vi "Encoders 1 SUBVI.vi"   [LabVIEW 2011]
uses:
  Robot Global Data.vi
types:
  T1 = typedef "WPI_RobotDriveDevRef.ctl" = cluster{"DevStatus":errorcluster, "Motors[]":T2[], "Square Inputs":bool, "Max Output":dbl, "Isochronous":bool}
  T2 = typedef "WPI_MotorControlDeviceRef.ctl" = cluster{"DeviceStatus":errorcluster, "Type":enum16{"PWM", "CAN"}, "PWM":cluster{"Digital Module":T3, "PWM Channel":T4, "DeadBand":T5}, "CAN":cluster{"Device Number":u8, "Control Mode":T6, "Semaphore":T7, "Max Vout":dbl}, "Invert":bool, "TransformRef":T8, "InvTransformRef":T8}
  T3 = typedef "FPGA_TypedefDigitalModule.ctl" = enum16{"Digital Module 1", "Digital Module 2"}
  T4 = typedef "FPGA_DIOPWMChannel.ctl" = enum8{"PWM 1", "PWM 2", "PWM 3", "PWM 4", "PWM 5", "PWM 6", "PWM 7", "PWM 8", "PWM 9", "PWM 10", "Invalid"}
  T5 = typedef "WPI_PWMDeadband.ctl" = cluster{"Name":string, "maxPositivePwm":i32, "minPositivePwm":i32, "centerPwm":i32, "maxNegativePwm":i32, "minNegativePwm":i32, "angularRange":u16}
  T6 = typedef "WPI_CANJaguar_ControlMode.ctl" = enum8{"Percent VBus", "Current", "Speed", "Position", "Voltage"}
  T7 = typedef "Semaphore RefNum" = refnum<k1>
  T8 = typedef "WPI_PWMTransform_ConPane.ctl" = refnum<vi>
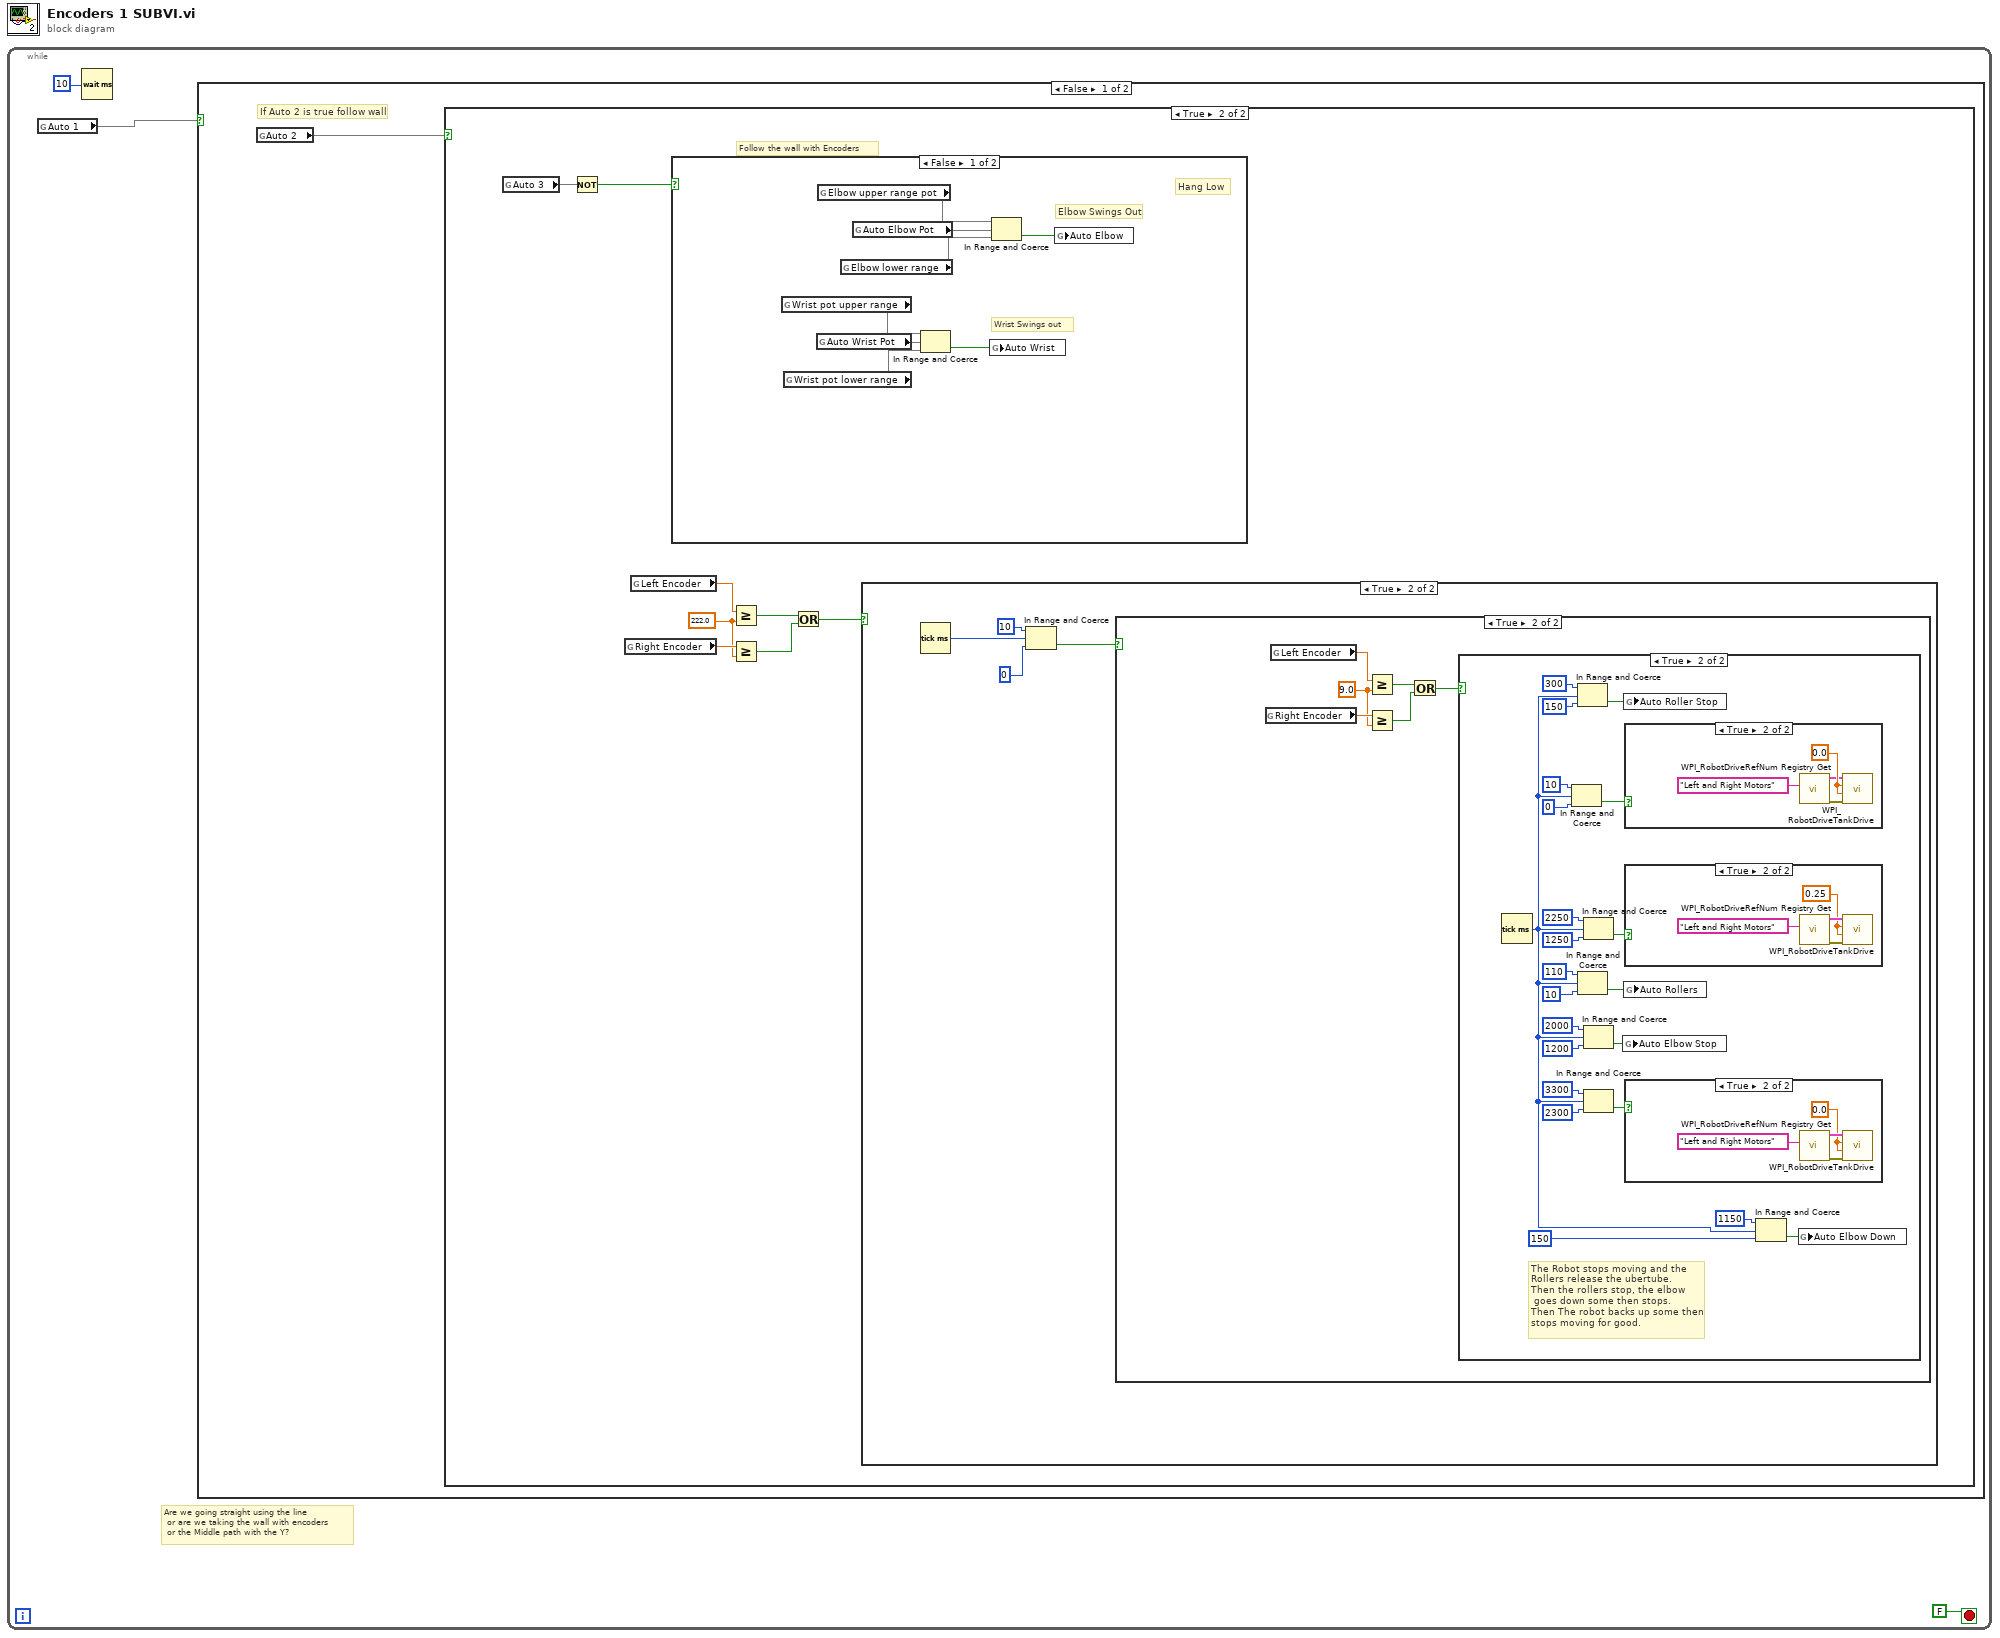
[diagram p0: block diagram]
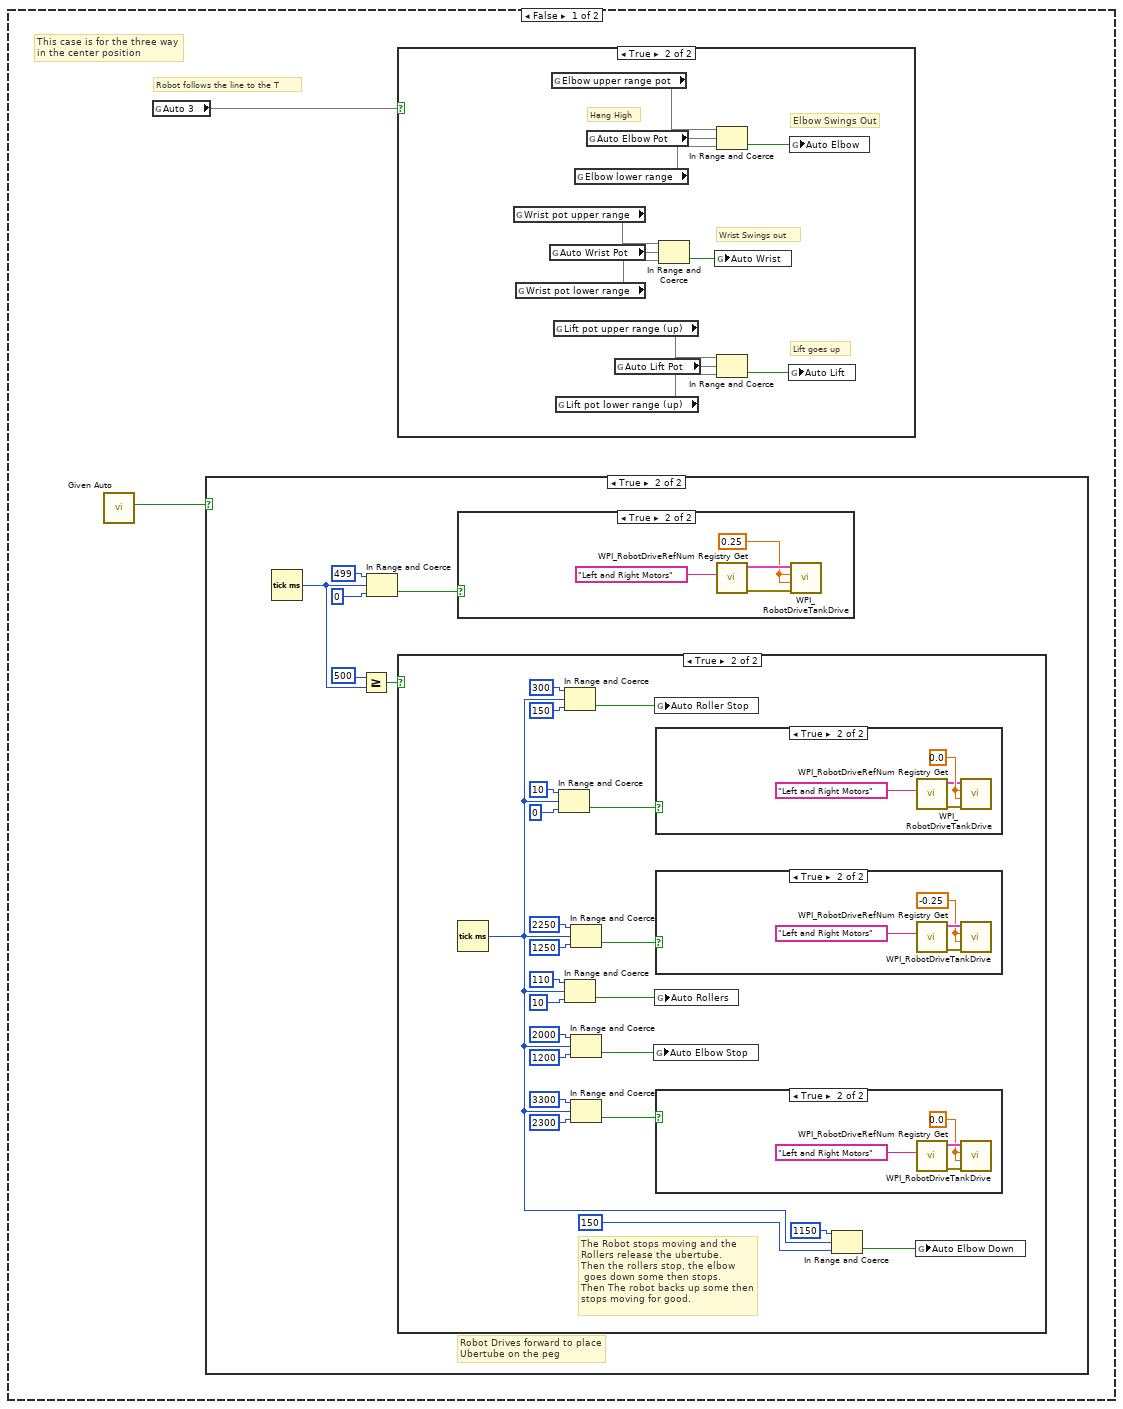
[diagram p2: hidden frame]
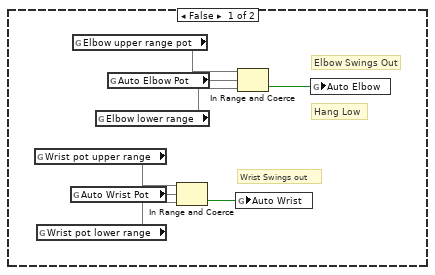
[diagram p9: hidden frame]
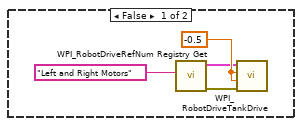
[diagram p10: hidden frame]
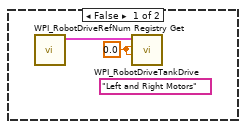
[diagram p11: hidden frame]
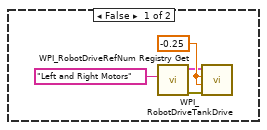
[diagram p12: hidden frame]
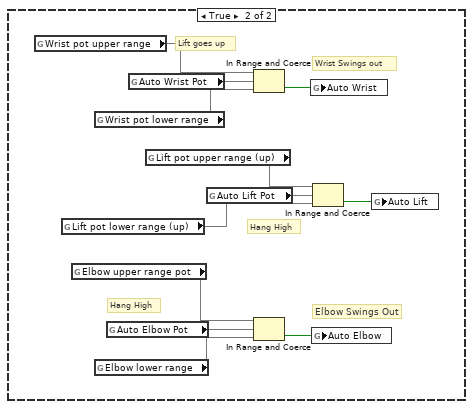
[diagram p16: hidden frame]
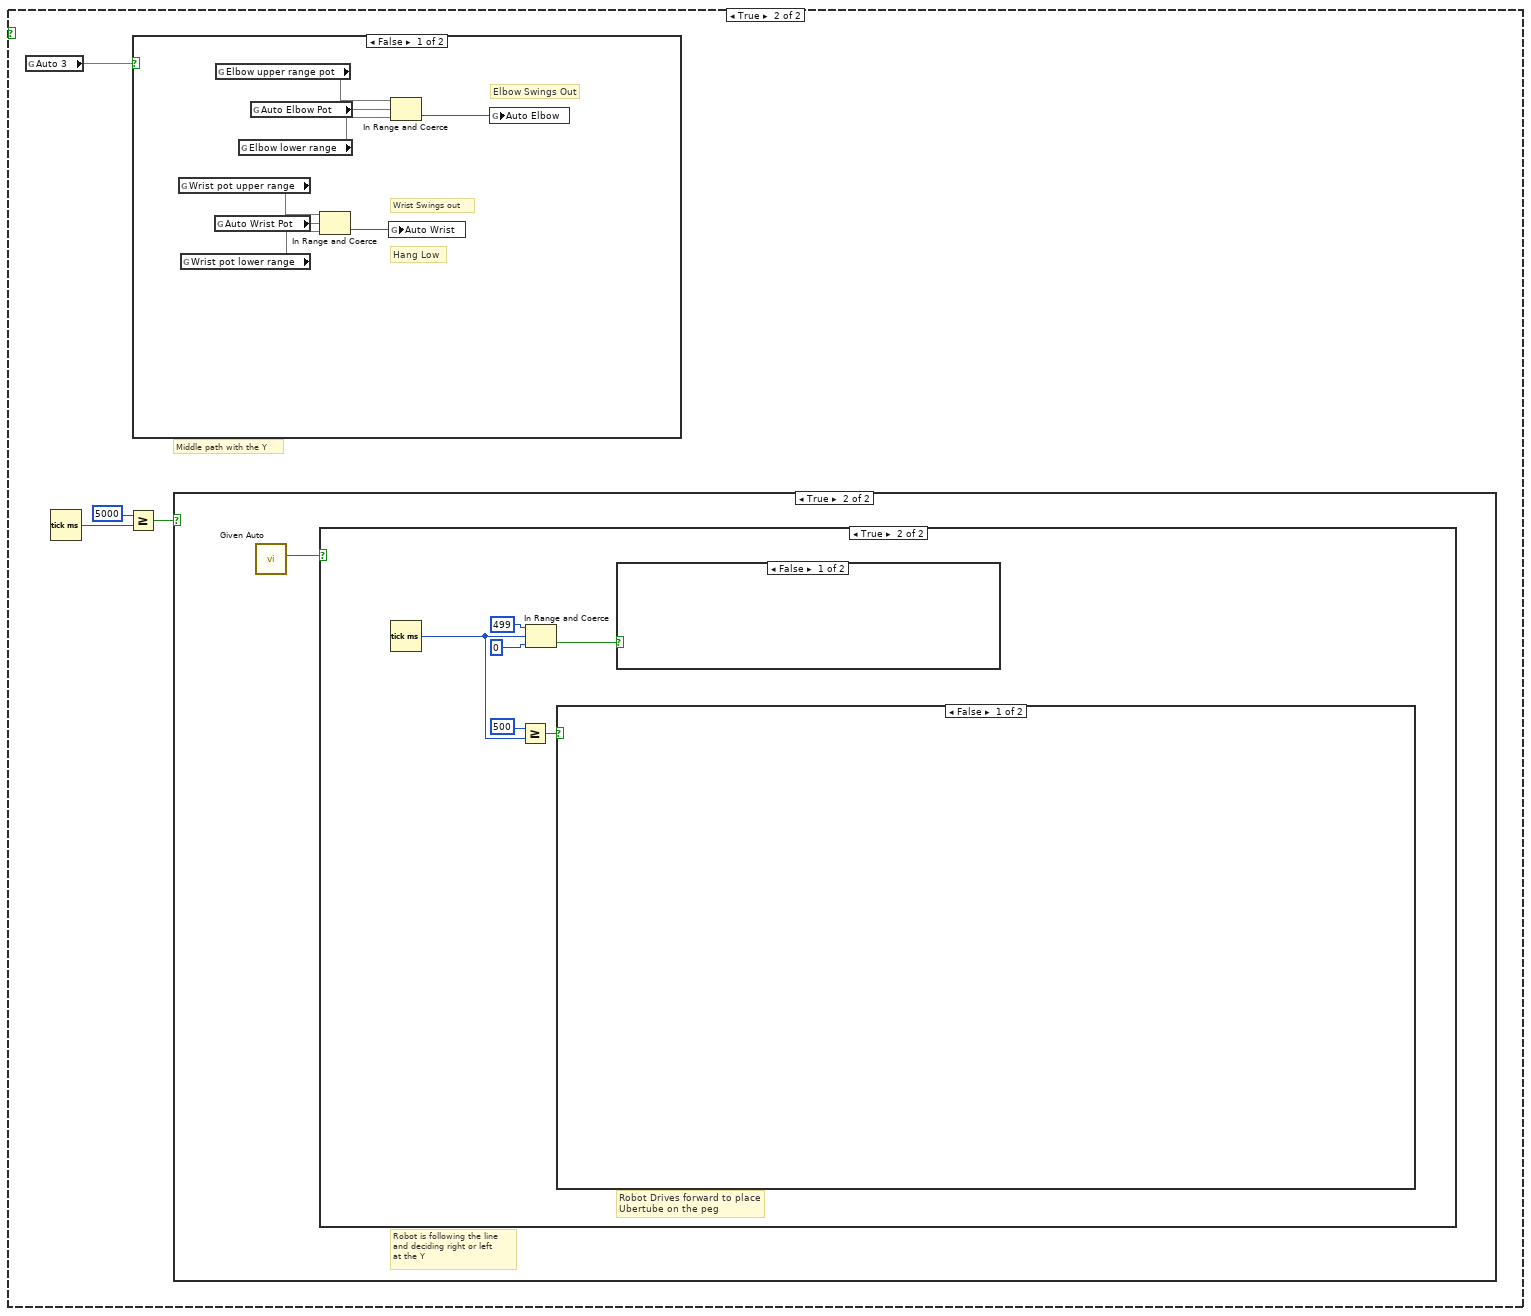
[diagram p17: hidden frame]
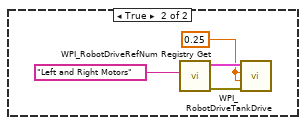
[diagram p20: hidden frame]
diagram:
  n1 = while {
    stop <- FALSE stop-if-true
    # "Are we going straight using the line\n or are we taking the wall with encoders\n or the Middle path with the Y?"
    n2 = global read "Robot Global Data.vi" "Auto 1"() -> (w1)
    n3 = Wait (ms)(milliseconds to wait=u32 10) -> ()  [unwired: 1 out]
    n4 = case shown="False" w1 {
      frame False {
        # "If Auto 2 is true follow wall"
        n5 = global read "Robot Global Data.vi" "Auto 2"() -> (w4)
        n6 = case shown="True" w4 {
          frame False {
            # "Robot follows the line to the T"
            # "This case is for the three way \nin the center position"
            n7 = call "Given Auto.vi"() -> ("x .or. y?"=w6:bool)  [unwired: 11 out]
            n8 = global read "Robot Global Data.vi" "Auto 3"() -> (w5)
            n9 = case shown="True" w6 {
              frame False {
              }
              frame True {
                # "Robot Drives forward to place\nUbertube on the peg"
                n10 = Tick Count (ms)() -> (millisecond timer value=w9:u32)
                n11 = Greater Or Equal?(x=u32 500, y=w9) -> (x >= y?=w11:bool)
                n12 = In Range and Coerce(upper limit=u32 499, x=w9, lower limit=u32 0) -> (In Range?=w10:bool)  [unwired: 1 out]
                n13 = case shown="True" w11 {
                  frame False {
                  }
                  frame True {
                    # "The Robot stops moving and the \nRollers release the ubertube. \nThen the rollers stop, the elbow\n goes down some then stops. \nThen The robot backs up some then \nstops moving for good."
                    n14 = Tick Count (ms)() -> (millisecond timer value=w17:u32)
                    n15 = In Range and Coerce(upper limit=u32 10, x=w17, lower limit=u32 0 ("x")) -> (In Range?=w18:bool)  [unwired: 1 out]
                    n16 = In Range and Coerce(upper limit=u32 300, x=w17, lower limit=u32 150 ("x")) -> (In Range?=w36:bool)  [unwired: 1 out]
                    n17 = In Range and Coerce(upper limit=u32 110, x=w17, lower limit=u32 10 ("x")) -> (In Range?=w38:bool)  [unwired: 1 out]
                    n18 = In Range and Coerce(upper limit=u32 2250, x=w17, lower limit=u32 1250 ("x")) -> (In Range?=w34:bool)  [unwired: 1 out]
                    n19 = In Range and Coerce(upper limit=u32 2000, x=w17, lower limit=u32 1200) -> (In Range?=w35:bool)  [unwired: 1 out]
                    n20 = In Range and Coerce(upper limit=u32 3300, x=w17, lower limit=u32 2300 ("x")) -> (In Range?=w33:bool)  [unwired: 1 out]
                    n21 = global write "Robot Global Data.vi" "Auto Elbow Stop"(w35) -> ()
                    n22 = global write "Robot Global Data.vi" "Auto Roller Stop"(w36) -> ()
                    n23 = global write "Robot Global Data.vi" "Auto Rollers"(w38) -> ()
                    n24 = case shown="True" w18 {
                      frame False {
                      }
                      frame True {
                        w42 = 0.0 ("Left axis value")
                        n25 = call <vilib>:"WPI_RobotDriveRefNum Registry Get.vi"("refnum name"="Left and Right Motors") -> ("error out"=w40:errorcluster, "RobotDriveDevRef"=w41:T1)  [unwired: 1 in, 8 out]
                        n26 = call <vilib>:"WPI_RobotDriveTankDrive.vi"("error in (no error)"=w40, "Right axis value"=w42, "Left axis value"=w42, "RobotDriveDevRef"=w41) -> ()  [unwired: 8 out]
                      }
                    }
                    n27 = case shown="True" w34 {
                      frame False {
                      }
                      frame True {
                        w47 = -0.25 ("Left axis value")
                        n28 = call <vilib>:"WPI_RobotDriveRefNum Registry Get.vi"("refnum name"="Left and Right Motors") -> ("error out"=w49:errorcluster, "RobotDriveDevRef"=w48:T1)  [unwired: 1 in, 8 out]
                        n29 = call <vilib>:"WPI_RobotDriveTankDrive.vi"("error in (no error)"=w49, "Right axis value"=w47, "Left axis value"=w47, "RobotDriveDevRef"=w48) -> ()  [unwired: 8 out]
                      }
                    }
                    n30 = case shown="True" w33 {
                      frame False {
                      }
                      frame True {
                        w43 = 0.0 ("Left axis value")
                        n31 = call <vilib>:"WPI_RobotDriveRefNum Registry Get.vi"("refnum name"="Left and Right Motors") -> ("error out"=w45:errorcluster, "RobotDriveDevRef"=w44:T1)  [unwired: 1 in, 8 out]
                        n32 = call <vilib>:"WPI_RobotDriveTankDrive.vi"("error in (no error)"=w45, "Right axis value"=w43, "Left axis value"=w43, "RobotDriveDevRef"=w44) -> ()  [unwired: 8 out]
                      }
                    }
                    n33 = In Range and Coerce(upper limit=u32 1150, x=w17, lower limit=u32 150 ("x")) -> (In Range?=w37:bool)  [unwired: 1 out]
                    n34 = global write "Robot Global Data.vi" "Auto Elbow Down"(w37) -> ()
                  }
                }
                n35 = case shown="True" w10 {
                  frame False {
                  }
                  frame True {
                    w13 = 0.25 ("Left axis value")
                    n36 = call <vilib>:"WPI_RobotDriveRefNum Registry Get.vi"("refnum name"="Left and Right Motors") -> ("error out"=w15:errorcluster, "RobotDriveDevRef"=w14:T1)  [unwired: 1 in, 8 out]
                    n37 = call <vilib>:"WPI_RobotDriveTankDrive.vi"("error in (no error)"=w15, "Right axis value"=w13, "Left axis value"=w13, "RobotDriveDevRef"=w14) -> ()  [unwired: 8 out]
                  }
                }
              }
            }
            n38 = case shown="True" w5 {
              frame False {
                # "Elbow Swings Out"
                # "Wrist Swings out"
                # "Hang Low"
                n39 = global read "Robot Global Data.vi" "Wrist pot upper range"() -> (w52)
                n40 = global read "Robot Global Data.vi" "Wrist pot lower range"() -> (w51)
                n41 = global read "Robot Global Data.vi" "Auto Wrist Pot"() -> (w57)
                n42 = global read "Robot Global Data.vi" "Elbow upper range pot"() -> (w54)
                n43 = global read "Robot Global Data.vi" "Elbow lower range"() -> (w53)
                n44 = global read "Robot Global Data.vi" "Auto Elbow Pot"() -> (w55)
                n45 = In Range and Coerce(upper limit=w52, x=w57, lower limit=w51) -> (In Range?=w58:bool)  [unwired: 1 out]
                n46 = global write "Robot Global Data.vi" "Auto Wrist"(w58) -> ()
                n47 = In Range and Coerce(upper limit=w54, x=w55, lower limit=w53) -> (In Range?=w56:bool)  [unwired: 1 out]
                n48 = global write "Robot Global Data.vi" "Auto Elbow"(w56) -> ()
              }
              frame True {
                # "Wrist Swings out"
                # "Elbow Swings Out"
                # "Lift goes up"
                # "Hang High"
                n49 = global read "Robot Global Data.vi" "Wrist pot upper range"() -> (w62)
                n50 = global read "Robot Global Data.vi" "Wrist pot lower range"() -> (w61)
                n51 = global read "Robot Global Data.vi" "Auto Wrist Pot"() -> (w66)
                n52 = global read "Robot Global Data.vi" "Elbow upper range pot"() -> (w60)
                n53 = global read "Robot Global Data.vi" "Lift pot upper range (up)"() -> (w64)
                n54 = global read "Robot Global Data.vi" "Lift pot lower range (up)"() -> (w63)
                n55 = global read "Robot Global Data.vi" "Elbow lower range"() -> (w59)
                n56 = global read "Robot Global Data.vi" "Auto Elbow Pot"() -> (w69)
                n57 = global read "Robot Global Data.vi" "Auto Lift Pot"() -> (w70)
                n58 = In Range and Coerce(upper limit=w62, x=w66, lower limit=w61) -> (In Range?=w65:bool)  [unwired: 1 out]
                n59 = global write "Robot Global Data.vi" "Auto Wrist"(w65) -> ()
                n60 = In Range and Coerce(upper limit=w60, x=w69, lower limit=w59) -> (In Range?=w68:bool)  [unwired: 1 out]
                n61 = In Range and Coerce(upper limit=w64, x=w70, lower limit=w63) -> (In Range?=w67:bool)  [unwired: 1 out]
                n62 = global write "Robot Global Data.vi" "Auto Lift"(w67) -> ()
                n63 = global write "Robot Global Data.vi" "Auto Elbow"(w68) -> ()
              }
            }
          }
          frame True {
            w74 = 222.0 ("y")
            # "Follow the wall with Encoders"
            n64 = global read "Robot Global Data.vi" "Auto 3"() -> (w78)
            n65 = Not(x=w78) -> (.not. x?=w77:bool)
            n66 = global read "Robot Global Data.vi" "Right Encoder"() -> (w75:dbl)
            n67 = global read "Robot Global Data.vi" "Left Encoder"() -> (w76:dbl)
            n68 = case shown="False" w77 {
              frame False {
                # "Elbow Swings Out"
                # "Wrist Swings out"
                # "Hang Low"
                n69 = global read "Robot Global Data.vi" "Wrist pot upper range"() -> (w134)
                n70 = global read "Robot Global Data.vi" "Wrist pot lower range"() -> (w133)
                n71 = global read "Robot Global Data.vi" "Auto Wrist Pot"() -> (w139)
                n72 = global read "Robot Global Data.vi" "Elbow upper range pot"() -> (w136)
                n73 = global read "Robot Global Data.vi" "Elbow lower range"() -> (w135)
                n74 = global read "Robot Global Data.vi" "Auto Elbow Pot"() -> (w137)
                n75 = In Range and Coerce(upper limit=w134, x=w139, lower limit=w133) -> (In Range?=w140:bool)  [unwired: 1 out]
                n76 = global write "Robot Global Data.vi" "Auto Wrist"(w140) -> ()
                n77 = In Range and Coerce(upper limit=w136, x=w137, lower limit=w135) -> (In Range?=w138:bool)  [unwired: 1 out]
                n78 = global write "Robot Global Data.vi" "Auto Elbow"(w138) -> ()
              }
              frame True {
                # "Hang High"
                # "Wrist Swings out"
                # "Elbow Swings Out"
                # "Lift goes up"
                # "Hang High"
                n79 = global read "Robot Global Data.vi" "Wrist pot upper range"() -> (w144)
                n80 = global read "Robot Global Data.vi" "Lift pot lower range (up)"() -> (w141)
                n81 = global read "Robot Global Data.vi" "Elbow upper range pot"() -> (w146)
                n82 = global read "Robot Global Data.vi" "Wrist pot lower range"() -> (w143)
                n83 = global read "Robot Global Data.vi" "Elbow lower range"() -> (w145)
                n84 = global read "Robot Global Data.vi" "Auto Elbow Pot"() -> (w151)
                n85 = global read "Robot Global Data.vi" "Auto Wrist Pot"() -> (w148)
                n86 = global read "Robot Global Data.vi" "Lift pot upper range (up)"() -> (w142)
                n87 = global read "Robot Global Data.vi" "Auto Lift Pot"() -> (w152)
                n88 = In Range and Coerce(upper limit=w144, x=w148, lower limit=w143) -> (In Range?=w147:bool)  [unwired: 1 out]
                n89 = In Range and Coerce(upper limit=w146, x=w151, lower limit=w145) -> (In Range?=w150:bool)  [unwired: 1 out]
                n90 = global write "Robot Global Data.vi" "Auto Wrist"(w147) -> ()
                n91 = global write "Robot Global Data.vi" "Auto Elbow"(w150) -> ()
                n92 = In Range and Coerce(upper limit=w142, x=w152, lower limit=w141) -> (In Range?=w149:bool)  [unwired: 1 out]
                n93 = global write "Robot Global Data.vi" "Auto Lift"(w149) -> ()
              }
            }
            n94 = Greater Or Equal?(x=w76, y=w74) -> (x >= y?=w73:bool)
            n95 = Greater Or Equal?(x=w75, y=w74) -> (x >= y?=w72:bool)
            n96 = Or(x=w73, y=w72) -> (x .or. y?=w71:bool)
            n97 = case shown="True" w71 {
              frame False {
                w82 = -0.5 ("Left axis value")
                n98 = call <vilib>:"WPI_RobotDriveRefNum Registry Get.vi"("refnum name"="Left and Right Motors") -> ("error out"=w80:errorcluster, "RobotDriveDevRef"=w81:T1)  [unwired: 1 in, 8 out]
                n99 = call <vilib>:"WPI_RobotDriveTankDrive.vi"("error in (no error)"=w80, "Right axis value"=w82, "Left axis value"=w82, "RobotDriveDevRef"=w81) -> ()  [unwired: 8 out]
              }
              frame True {
                n100 = Tick Count (ms)() -> (millisecond timer value=w83:u32)
                n101 = In Range and Coerce(upper limit=u32 10, x=w83, lower limit=u32 0 ("millisecond timer value")) -> (In Range?=w85:bool)  [unwired: 1 out]
                n102 = case shown="True" w85 {
                  frame False {
                    w87 = 0.0 ("Left axis value")
                    (unwired) "Left and Right Motors" ("refnum name")
                    n103 = call <vilib>:"WPI_RobotDriveRefNum Registry Get.vi"() -> ("RobotDriveDevRef"=w88:T1)  [unwired: 2 in, 9 out]
                    n104 = call <vilib>:"WPI_RobotDriveTankDrive.vi"("Right axis value"=w87, "Left axis value"=w87, "RobotDriveDevRef"=w88) -> ()  [unwired: 1 in, 8 out]
                  }
                  frame True {
                    w92 = 9.0 ("y")
                    n105 = global read "Robot Global Data.vi" "Right Encoder"() -> (w93:dbl)
                    n106 = global read "Robot Global Data.vi" "Left Encoder"() -> (w94:dbl)
                    n107 = Greater Or Equal?(x=w94, y=w92) -> (x >= y?=w91:bool)
                    n108 = Greater Or Equal?(x=w93, y=w92) -> (x >= y?=w90:bool)
                    n109 = Or(x=w91, y=w90) -> (x .or. y?=w89:bool)
                    n110 = case shown="True" w89 {
                      frame False {
                        w98 = -0.25 ("Left axis value")
                        n111 = call <vilib>:"WPI_RobotDriveRefNum Registry Get.vi"("refnum name"="Left and Right Motors") -> ("error out"=w96:errorcluster, "RobotDriveDevRef"=w97:T1)  [unwired: 1 in, 8 out]
                        n112 = call <vilib>:"WPI_RobotDriveTankDrive.vi"("error in (no error)"=w96, "Right axis value"=w98, "Left axis value"=w98, "RobotDriveDevRef"=w97) -> ()  [unwired: 8 out]
                      }
                      frame True {
                        # "The Robot stops moving and the \nRollers release the ubertube. \nThen the rollers stop, the elbow\n goes down some then stops. \nThen The robot backs up some then \nstops moving for good."
                        n113 = Tick Count (ms)() -> (millisecond timer value=w99:u32)
                        n114 = In Range and Coerce(upper limit=u32 10, x=w99, lower limit=u32 0 ("x")) -> (In Range?=w100:bool)  [unwired: 1 out]
                        n115 = In Range and Coerce(upper limit=u32 300, x=w99, lower limit=u32 150 ("x")) -> (In Range?=w118:bool)  [unwired: 1 out]
                        n116 = In Range and Coerce(upper limit=u32 110, x=w99, lower limit=u32 10 ("x")) -> (In Range?=w120:bool)  [unwired: 1 out]
                        n117 = In Range and Coerce(upper limit=u32 2250, x=w99, lower limit=u32 1250 ("x")) -> (In Range?=w116:bool)  [unwired: 1 out]
                        n118 = In Range and Coerce(upper limit=u32 2000, x=w99, lower limit=u32 1200) -> (In Range?=w117:bool)  [unwired: 1 out]
                        n119 = In Range and Coerce(upper limit=u32 3300, x=w99, lower limit=u32 2300 ("x")) -> (In Range?=w115:bool)  [unwired: 1 out]
                        n120 = global write "Robot Global Data.vi" "Auto Elbow Stop"(w117) -> ()
                        n121 = global write "Robot Global Data.vi" "Auto Roller Stop"(w118) -> ()
                        n122 = global write "Robot Global Data.vi" "Auto Rollers"(w120) -> ()
                        n123 = case shown="True" w100 {
                          frame False {
                          }
                          frame True {
                            w124 = 0.0 ("Left axis value")
                            n124 = call <vilib>:"WPI_RobotDriveRefNum Registry Get.vi"("refnum name"="Left and Right Motors") -> ("error out"=w122:errorcluster, "RobotDriveDevRef"=w123:T1)  [unwired: 1 in, 8 out]
                            n125 = call <vilib>:"WPI_RobotDriveTankDrive.vi"("error in (no error)"=w122, "Right axis value"=w124, "Left axis value"=w124, "RobotDriveDevRef"=w123) -> ()  [unwired: 8 out]
                          }
                        }
                        n126 = case shown="True" w116 {
                          frame False {
                          }
                          frame True {
                            w129 = 0.25 ("Left axis value")
                            n127 = call <vilib>:"WPI_RobotDriveRefNum Registry Get.vi"("refnum name"="Left and Right Motors") -> ("error out"=w131:errorcluster, "RobotDriveDevRef"=w130:T1)  [unwired: 1 in, 8 out]
                            n128 = call <vilib>:"WPI_RobotDriveTankDrive.vi"("error in (no error)"=w131, "Right axis value"=w129, "Left axis value"=w129, "RobotDriveDevRef"=w130) -> ()  [unwired: 8 out]
                          }
                        }
                        n129 = case shown="True" w115 {
                          frame False {
                          }
                          frame True {
                            w125 = 0.0 ("Left axis value")
                            n130 = call <vilib>:"WPI_RobotDriveRefNum Registry Get.vi"("refnum name"="Left and Right Motors") -> ("error out"=w127:errorcluster, "RobotDriveDevRef"=w126:T1)  [unwired: 1 in, 8 out]
                            n131 = call <vilib>:"WPI_RobotDriveTankDrive.vi"("error in (no error)"=w127, "Right axis value"=w125, "Left axis value"=w125, "RobotDriveDevRef"=w126) -> ()  [unwired: 8 out]
                          }
                        }
                        n132 = In Range and Coerce(upper limit=u32 1150, x=w99, lower limit=u32 150 ("x")) -> (In Range?=w119:bool)  [unwired: 1 out]
                        n133 = global write "Robot Global Data.vi" "Auto Elbow Down"(w119) -> ()
                      }
                    }
                  }
                }
              }
            }
          }
        }
      }
      frame True {
        # "Middle path with the Y"
        n134 = global read "Robot Global Data.vi" "Auto 3"() -> (w153)
        n135 = Tick Count (ms)() -> (millisecond timer value=w156:u32)
        n136 = Greater Or Equal?(x=u32 5000, y=w156) -> (x >= y?=w154:bool)
        n137 = case shown="False" w153 {
          frame False {
            # "Elbow Swings Out"
            # "Wrist Swings out"
            # "Hang Low"
            n138 = global read "Robot Global Data.vi" "Wrist pot upper range"() -> (w201)
            n139 = global read "Robot Global Data.vi" "Wrist pot lower range"() -> (w199)
            n140 = global read "Robot Global Data.vi" "Auto Wrist Pot"() -> (w200)
            n141 = global read "Robot Global Data.vi" "Elbow upper range pot"() -> (w203)
            n142 = global read "Robot Global Data.vi" "Elbow lower range"() -> (w202)
            n143 = global read "Robot Global Data.vi" "Auto Elbow Pot"() -> (w204)
            n144 = In Range and Coerce(upper limit=w201, x=w200, lower limit=w199) -> (In Range?=w206:bool)  [unwired: 1 out]
            n145 = global write "Robot Global Data.vi" "Auto Wrist"(w206) -> ()
            n146 = In Range and Coerce(upper limit=w203, x=w204, lower limit=w202) -> (In Range?=w205:bool)  [unwired: 1 out]
            n147 = global write "Robot Global Data.vi" "Auto Elbow"(w205) -> ()
          }
          frame True {
            # "Wrist Swings out"
            # "Elbow Swings Out"
            # "Lift goes up"
            # "Hang High"
            n148 = global read "Robot Global Data.vi" "Wrist pot upper range"() -> (w211)
            n149 = global read "Robot Global Data.vi" "Elbow upper range pot"() -> (w213)
            n150 = global read "Robot Global Data.vi" "Lift pot upper range (up)"() -> (w208)
            n151 = global read "Robot Global Data.vi" "Lift pot lower range (up)"() -> (w207)
            n152 = global read "Robot Global Data.vi" "Wrist pot lower range"() -> (w209)
            n153 = global read "Robot Global Data.vi" "Auto Wrist Pot"() -> (w210)
            n154 = global read "Robot Global Data.vi" "Auto Lift Pot"() -> (w218)
            n155 = global read "Robot Global Data.vi" "Elbow lower range"() -> (w212)
            n156 = global read "Robot Global Data.vi" "Auto Elbow Pot"() -> (w217)
            n157 = In Range and Coerce(upper limit=w211, x=w210, lower limit=w209) -> (In Range?=w214:bool)  [unwired: 1 out]
            n158 = In Range and Coerce(upper limit=w208, x=w218, lower limit=w207) -> (In Range?=w215:bool)  [unwired: 1 out]
            n159 = global write "Robot Global Data.vi" "Auto Wrist"(w214) -> ()
            n160 = global write "Robot Global Data.vi" "Auto Lift"(w215) -> ()
            n161 = In Range and Coerce(upper limit=w213, x=w217, lower limit=w212) -> (In Range?=w216:bool)  [unwired: 1 out]
            n162 = global write "Robot Global Data.vi" "Auto Elbow"(w216) -> ()
          }
        }
        n163 = case shown="True" w154 {
          frame False {
          }
          frame True {
            # "Robot is following the line\nand deciding right or left\nat the Y"
            n164 = call "Given Auto.vi"() -> ("x .or. y?"=w157:bool)  [unwired: 11 out]
            n165 = case shown="True" w157 {
              frame False {
              }
              frame True {
                # "Robot Drives forward to place\nUbertube on the peg"
                n166 = Tick Count (ms)() -> (millisecond timer value=w160:u32)
                n167 = Greater Or Equal?(x=u32 500, y=w160) -> (x >= y?=w162:bool)
                n168 = In Range and Coerce(upper limit=u32 499, x=w160, lower limit=u32 0) -> (In Range?=w161:bool)  [unwired: 1 out]
                n169 = case shown="False" w162 {
                  frame False {
                  }
                  frame True {
                    w190 = 0.0 ("Left axis value")
                    # "The Robot stops moving and the \nRollers release the ubertube. \nThen the rollers stop, the elbow\n goes down some then stops. \nThen The robot backs up some then \nstops moving for good."
                    n170 = Tick Count (ms)() -> (millisecond timer value=w169:u32)
                    n171 = call <vilib>:"WPI_RobotDriveRefNum Registry Get.vi"("refnum name"="Left and Right Motors") -> ("error out"=w188:errorcluster, "RobotDriveDevRef"=w189:T1)  [unwired: 1 in, 8 out]
                    n172 = call <vilib>:"WPI_RobotDriveTankDrive.vi"("error in (no error)"=w188, "Right axis value"=w190, "Left axis value"=w190, "RobotDriveDevRef"=w189) -> ()  [unwired: 8 out]
                    n173 = In Range and Coerce(upper limit=u32 300, x=w169, lower limit=u32 150 ("x")) -> (In Range?=w184:bool)  [unwired: 1 out]
                    n174 = In Range and Coerce(upper limit=u32 110, x=w169, lower limit=u32 10 ("x")) -> (In Range?=w186:bool)  [unwired: 1 out]
                    n175 = In Range and Coerce(upper limit=u32 2250, x=w169, lower limit=u32 1250 ("x")) -> (In Range?=w182:bool)  [unwired: 1 out]
                    n176 = In Range and Coerce(upper limit=u32 2000, x=w169, lower limit=u32 1200) -> (In Range?=w183:bool)  [unwired: 1 out]
                    n177 = In Range and Coerce(upper limit=u32 3300, x=w169, lower limit=u32 2300 ("x")) -> (In Range?=w181:bool)  [unwired: 1 out]
                    n178 = In Range and Coerce(upper limit=u32 1150, x=w169, lower limit=u32 150 ("x")) -> (In Range?=w185:bool)  [unwired: 1 out]
                    n179 = global write "Robot Global Data.vi" "Auto Elbow Stop"(w183) -> ()
                    n180 = global write "Robot Global Data.vi" "Auto Roller Stop"(w184) -> ()
                    n181 = global write "Robot Global Data.vi" "Auto Rollers"(w186) -> ()
                    n182 = global write "Robot Global Data.vi" "Auto Elbow Down"(w185) -> ()
                    n183 = case shown="True" w182 {
                      frame False {
                      }
                      frame True {
                        w195 = -0.25 ("Left axis value")
                        n184 = call <vilib>:"WPI_RobotDriveRefNum Registry Get.vi"("refnum name"="Left and Right Motors") -> ("error out"=w197:errorcluster, "RobotDriveDevRef"=w196:T1)  [unwired: 1 in, 8 out]
                        n185 = call <vilib>:"WPI_RobotDriveTankDrive.vi"("error in (no error)"=w197, "Right axis value"=w195, "Left axis value"=w195, "RobotDriveDevRef"=w196) -> ()  [unwired: 8 out]
                      }
                    }
                    n186 = case shown="True" w181 {
                      frame False {
                      }
                      frame True {
                        w191 = 0.0 ("Left axis value")
                        n187 = call <vilib>:"WPI_RobotDriveRefNum Registry Get.vi"("refnum name"="Left and Right Motors") -> ("error out"=w193:errorcluster, "RobotDriveDevRef"=w192:T1)  [unwired: 1 in, 8 out]
                        n188 = call <vilib>:"WPI_RobotDriveTankDrive.vi"("error in (no error)"=w193, "Right axis value"=w191, "Left axis value"=w191, "RobotDriveDevRef"=w192) -> ()  [unwired: 8 out]
                      }
                    }
                  }
                }
                n189 = case shown="False" w161 {
                  frame False {
                  }
                  frame True {
                    w164 = 0.25 ("Left axis value")
                    n190 = call <vilib>:"WPI_RobotDriveRefNum Registry Get.vi"("refnum name"="Left and Right Motors") -> ("error out"=w166:errorcluster, "RobotDriveDevRef"=w165:T1)  [unwired: 1 in, 8 out]
                    n191 = call <vilib>:"WPI_RobotDriveTankDrive.vi"("error in (no error)"=w166, "Right axis value"=w164, "Left axis value"=w164, "RobotDriveDevRef"=w165) -> ()  [unwired: 8 out]
                  }
                }
              }
            }
          }
        }
      }
    }
  }
